vi "Deconstruct.vi"(0 "iUser Configuration Manager DVR":refnum<data-value>, 11 "Error In":errorcluster) -> (15 "Error Out":errorcluster)   [LabVIEW 2017, in "User Configuration Manager.lvlib" / "By Ref.lvlib"]
uses:
  <vilib>/gpm_packages/@cs/user-manager/Source/User Configuration Manager Ref/By Ref.lvlib
  <vilib>/gpm_packages/@cs/user-manager/Source/iUser Configuration Manager/iUser Configuration Manager.lvclass
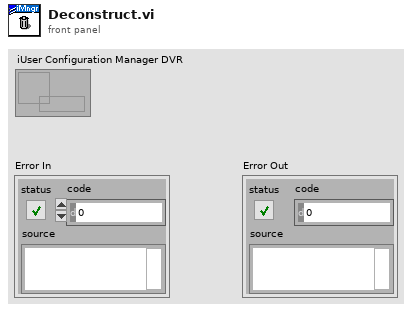
[diagram p1: front panel]
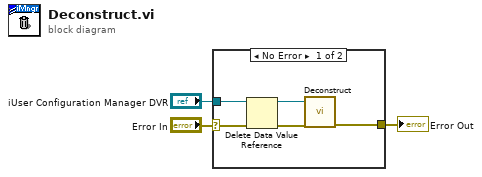
[diagram p0: block diagram]
diagram:
  n1 = case shown="No Error" "Error In" {
    selector: "Error In" -> [w5 w9]
    tunnel: [w8 w9] -> w1
    tunnel: "iUser Configuration Manager DVR" -> [w7 _]
    frame No Error {
      n2 = Delete Data Value Reference(data value reference=w7, error in=w5) -> (data value=w6:refnum<class "iUser Configuration Manager.lvclass">, error out=w4:errorcluster)
      n3 = call-dynamic "Deconstruct.vi"("iUser Configuration Manager in"=w6, "error in (no error)"=w4) -> ("error out"=w8:errorcluster)  [unwired: 13 in]
    }
    frame Error {
    }
  }
  "Error Out" <- w1
